vi "WC Stability.vi"(4 "Data In":cluster{"t0":dbl, "dt":dbl, "Y":dbl[]}={"t0"=0.0, "dt"=1.0, "Y"=[]} {"Y" min=0.0 max=127.0 format="%.2f"; "dt" format="%.3p"; "t0" format="%.2f"}) -> (1 "Stability":dbl format="%.6p")   [LabVIEW 2019]
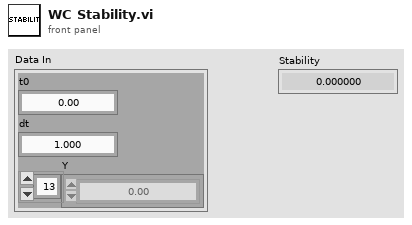
[diagram p1: front panel]
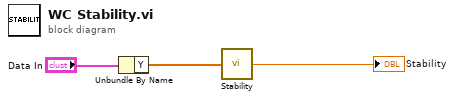
[diagram p0: block diagram]
diagram:
  n1 = Unbundle By Name("Data In") -> ("Y"=w2:dbl[])
  n2 = call "Stability.vi"("Array"=w2) -> ("Stability"=→"Stability":dbl)  [unwired: 4 in]
